vi "workspace_cache.get_from_rid.vi"(8 "error in":errorcluster, 10 "Workspace RID":string, 11 "Nominal Client in":refnum<class "Nominal Client.lvclass">) -> (0 "error out":errorcluster, 1 "Valid?":bool, 2 "Workspace":refnum<class "workspace.lvclass">, 3 "Nominal Client out":refnum<class "Nominal Client.lvclass">)   [LabVIEW 2020, in "Nominal Client.lvclass"]
uses:
  Nominal Client.lvclass
  Nominal Client.lvclass/Nominal Client.ctl
  nominal types/workspace/workspace.lvclass
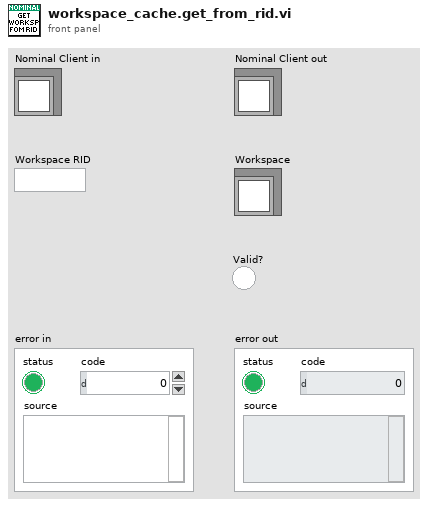
[diagram p1: front panel]
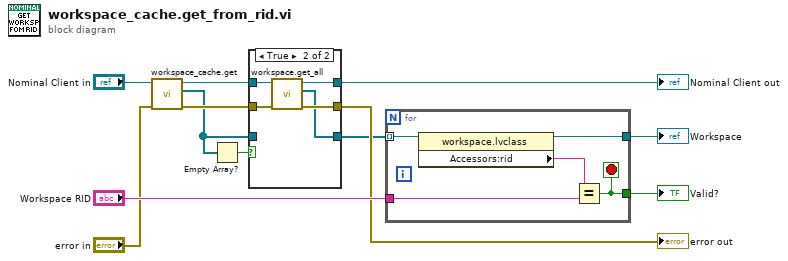
[diagram p0: block diagram]
diagram:
  n1 = call "workspace_cache.get.vi"("error in"="error in", "Nominal Client in"="Nominal Client in") -> ("error out"=w6:errorcluster, "Workspace"=w2:refnum<class "workspace.lvclass">[], "Nominal Client out"=w8:refnum<class "Nominal Client.lvclass">)  [unwired: 7 in]
  n2 = Empty Array?(array=w2) -> (empty?=w3:bool)
  n3 = case shown="True" w3 {
    tunnel: w8 -> [w14 w20]
    tunnel: w6 -> [w13 w19]
    tunnel: [w13 w18] -> w5
    tunnel: [w15 w17] -> w1
    tunnel: [w14 w16] -> w4
    tunnel: w2 -> [w15 _]
    frame False {
    }
    frame True {
      n4 = call "workspace.get_all.vi"("error in"=w19, "Nominal Client in"=w20) -> ("error out"=w18:errorcluster, "Workspaces"=w17:refnum<class "workspace.lvclass">[], "Nominal Client out"=w16:refnum<class "Nominal Client.lvclass">)  [unwired: 7 in]
    }
  }
  "Nominal Client out" <- w4
  "error out" <- w5
  n5 = for {
    tunnel: w1 -> [w25] mode=indexing
    tunnel: [w24] -> w11
    tunnel: "Workspace RID" -> [w22]
    tunnel: [w21] -> w10
    stop <- w21 stop-if-true
    n6 = property class="workspace.lvclass"(reference=w25) -> (reference out=w24:refnum<class "workspace.lvclass">, "Accessors:rid"=w23:string)  [unwired: 1 in, 1 out]
    n7 = Equal?(x=w23, y=w22) -> (x = y?=w21:bool)
  }
  "Workspace" <- w11
  "Valid?" <- w10
